vi "DBItemName-Log.vi"() -> (1 "Items":string[](array[string]))   [LabVIEW 2015, in "FileHandler.lvlib"]
uses:
  FileHandler.lvlib
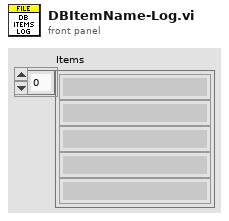
[diagram p1: front panel]
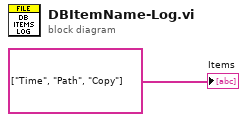
[diagram p0: block diagram]
diagram:
  "Items" <- string[] ["Time", "Path", "Copy"]
